vi "EOL CAN_Start_Teach.vi"(7 "Rx Arbitration Id":u32=402522244 format="%.0x", 8 "Error in":errorcluster, 9 "Glass?":bool, 10 "Read Session in":refnum<k21>, 11 "Write Session in":refnum<k21>) -> (0 "Error out":errorcluster, 2 "TxRx Data":string[][](array[string]), 3 "Response Good?":bool)   [LabVIEW 2015]
uses:
  <vilib>/xnet/xnet.llb/XNET Frame CAN.ctl
  <vilib>/xnet/xnet.llb/XNET Frame Type CAN.ctl
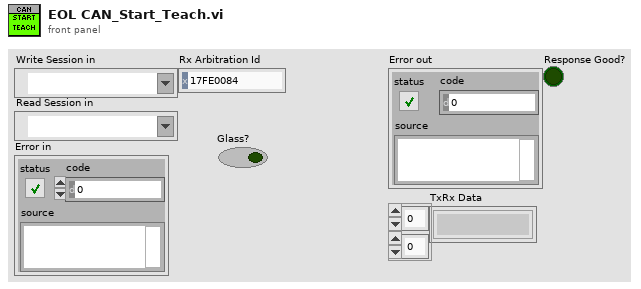
[diagram p1: front panel]
types:
  T1 = typedef "XNET Frame CAN.ctl" = cluster{"timestamp":timestamp, "payload":u8[], "identifier":u32, "type":T2, "extended?":bool, "echo?":bool}
  T2 = typedef "XNET Frame Type CAN.ctl" = u8
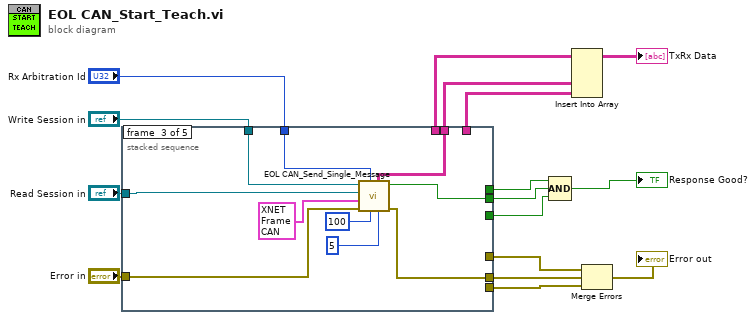
[diagram p0: block diagram]
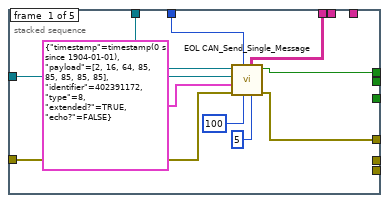
[diagram p2: hidden frame]
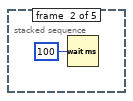
[diagram p3: hidden frame]
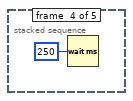
[diagram p4: hidden frame]
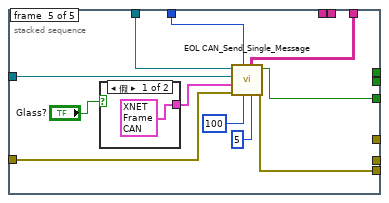
[diagram p5: hidden frame]
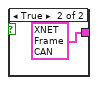
[diagram p6: hidden frame]
diagram:
  n1 = stacked-sequence {
    tunnel: "Error in" -> [w26 _ w34 _ w46]
    tunnel: "Read Session in" -> [w25 _ w36 _ w42]
    tunnel: "Write Session in" -> [w24 _ w35 _ w41]
    tunnel: "Rx Arbitration Id" -> [w23 _ w31 _ w40]
    tunnel: [w22 _ _ _ _] -> w3
    tunnel: [w21 _ _ _ _] -> w10
    tunnel: [_ _ _ _ w45] -> w6
    tunnel: [_ _ _ _ w44] -> w1
    tunnel: [w20 _ _ _ _] -> w8
    tunnel: [_ _ _ _ w43] -> w7
    tunnel: [_ _ w30 _ _] -> w2
    tunnel: [_ _ w29 _ _] -> w5
    tunnel: [_ _ w28 _ _] -> w4
    frame #0 {
      n2 = call <userlib>:"EOL CAN_Send_Single_Message.vi"("Retries"=5, "Msg Wait Time"=u32 100, "Rx Arbitration Id"=w23, "Error in"=w26, "Tx CAN frame"=T1 {"timestamp"=timestamp(0 s since 1904-01-01), "payload"=[2, 16, 64, 85, 85, 85, 85, 85], "identifier"=402391172, "type"=8, "extended?"=TRUE, "echo?"=FALSE}, "Read Session in"=w25, "Write Session in"=w24) -> ("Error out"=w20:errorcluster, "Response Good?"=w21:bool, "TxRx Data"=w22:string[][])  [unwired: 2 out]
    }
    frame #1 {
      n3 = Wait (ms)(milliseconds to wait=u32 100) -> ()  [unwired: 1 out]
    }
    frame #2 {
      n4 = call <userlib>:"EOL CAN_Send_Single_Message.vi"("Retries"=5, "Msg Wait Time"=u32 100, "Rx Arbitration Id"=w31, "Error in"=w34, "Tx CAN frame"=T1 {"timestamp"=timestamp(0 s since 1904-01-01), "payload"=[4, 46, 253, 17, 0, 85, 85, 85], "identifier"=402391172, "type"=8, "extended?"=TRUE, "echo?"=FALSE}, "Read Session in"=w36, "Write Session in"=w35) -> ("Error out"=w28:errorcluster, "Response Good?"=w29:bool, "TxRx Data"=w30:string[][])  [unwired: 2 out]
    }
    frame #3 {
      n5 = Wait (ms)(milliseconds to wait=u32 250) -> ()  [unwired: 1 out]
    }
    frame #4 {
      n6 = case shown="假" "Glass?" {
        tunnel: [T1 {"timestamp"=timestamp(0 s since 1904-01-01), "payload"=[7, 49, 1, 5, 36, 64, 0, 0], "identifier"=402391172, "type"=8, "extended?"=TRUE, "echo?"=FALSE} ("Tx CAN frame") T1 {"timestamp"=timestamp(0 s since 1904-01-01), "payload"=[7, 49, 1, 5, 35, 64, 0, 0], "identifier"=402391172, "type"=8, "extended?"=TRUE, "echo?"=FALSE} ("Tx CAN frame")] -> w47
        frame False {
        }
        frame True {
        }
      }
      n7 = call <userlib>:"EOL CAN_Send_Single_Message.vi"("Retries"=5, "Msg Wait Time"=u32 100, "Rx Arbitration Id"=w40, "Error in"=w46, "Tx CAN frame"=w47, "Read Session in"=w42, "Write Session in"=w41) -> ("Error out"=w43:errorcluster, "Response Good?"=w45:bool, "TxRx Data"=w44:string[][])  [unwired: 2 out]
    }
  }
  n8 = Compound Arithmetic op=AND(w10, w5, w6) -> (→"Response Good?":bool)
  n9 = Insert Into Array(array=w3, new element #1=w2, new element #2=w1) -> (→"TxRx Data":string[][])  [unwired: 2 in]
  n10 = Merge Errors(w8, w4, w7) -> (→"Error out":errorcluster)
